vi "项名.vi"(8 "error in (no error)":errorcluster caption="错误输入（无错误）", 11 "LNK 输入":refnum<class "Menu.lvclass">) -> (0 "error out":errorcluster caption="错误输出", 3 "LNK 输出":refnum<class "Menu.lvclass">)   [LabVIEW 2016, in "Menu.lvclass"]
uses:
  Menu.lvclass
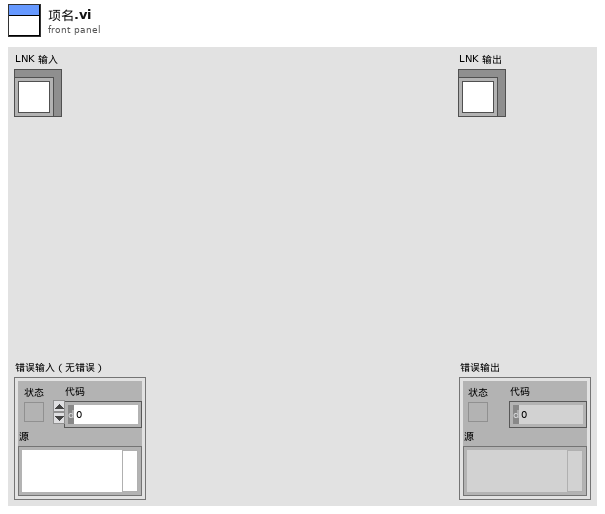
[diagram p1: front panel]
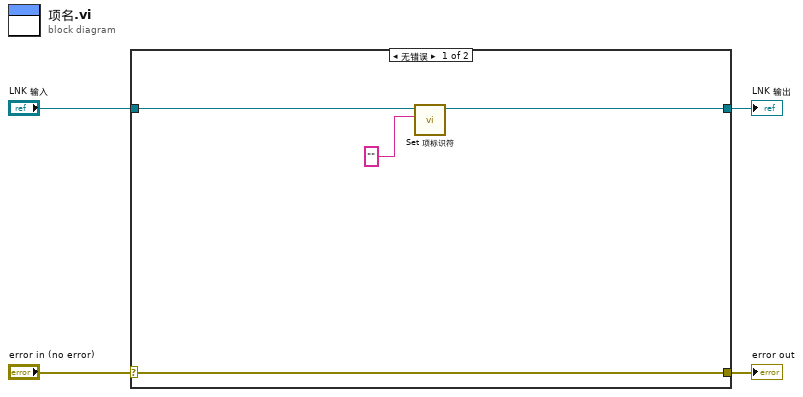
[diagram p0: block diagram]
diagram:
  n1 = case shown="无错误" "error in (no error)" {
    selector: "error in (no error)" -> [w7 w10]
    tunnel: [w7 w10] -> w3
    tunnel: [w6 w9] -> w1
    tunnel: "LNK 输入" -> [w8 w9]
    frame No Error {
      n2 = call "Set 项标识符.vi"("项标识符"="", "LNK in"=w8) -> ("LNK out"=w6:refnum<class "Menu.lvclass">)  [unwired: 9 in]
    }
    frame Error {
    }
  }
  "error out" <- w3
  "LNK 输出" <- w1
